vi "Telemetry.vi"   [LabVIEW 2018]
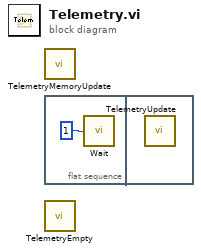
[diagram p0: block diagram]
diagram:
  n1 = call "TelemetryMemoryUpdate.vi"() -> ()  [unwired: 12 in]
  n2 = flat-sequence {
    frame #0 {
      n3 = call "Wait"("Count(mSec)"=u8 1) -> ()  [unwired: 1 out]
    }
    frame #1 {
      n4 = call "TelemetryUpdate.vi"() -> ()  [unwired: 12 in]
    }
  }
  n5 = call "TelemetryEmpty.vi"() -> ()  [unwired: 12 in]
